vi "GetTransconductanceIntensity.vi"(7 "LabVIEW Web Service Request":refnum<class "Web Request.lvclass">) -> ()   [LabVIEW 2016]
uses:
  <vilib>/wsapi/Web Request.lvclass
  <vilib>/wsapi/NI_WebServices.lvlib
panel:
  # "Use the Web Service Request input terminal to call the VIs on the Web Services palette. Do not remove it from the connector pane unless you don't need access to the palette."
  # "Each additional control wired to the connector pane will be available as an input in the URL. To include an indicator in terminal-mode output (the default setting), it must also be wired to the connector pane."
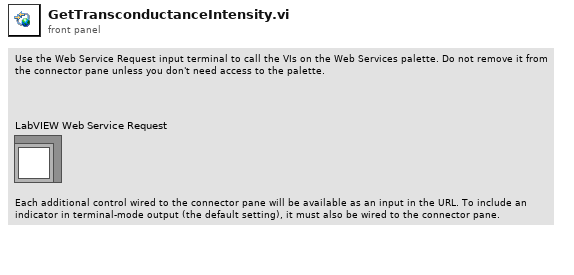
[diagram p1: front panel]
types:
  T1 = typedef "imagedata.ctl" = cluster{"image type":i32, "image depth":i32, "image":u8[], "mask":u8[], "colors":u32[], "Rectangle":cluster{"left":i16, "top":i16, "right":i16, "bottom":i16}}
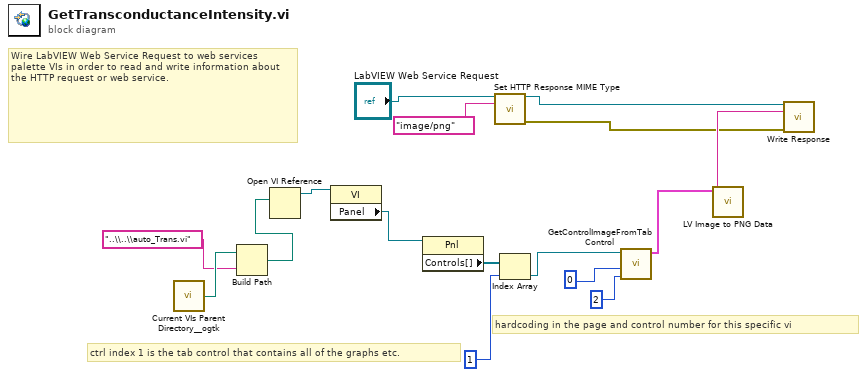
[diagram p0: block diagram]
diagram:
  # "hardcoding in the page and control number for this specific vi"
  # "ctrl index 1 is the tab control that contains all of the graphs etc."
  # "Wire LabVIEW Web Service Request to web services palette VIs in order to read and write information about the HTTP request or web service."
  n1 = call <userlib>:"Current VIs Parent Directory__ogtk.vi"() -> ("Parent Directory (+ Relative)"=w10:path)  [unwired: 5 in]
  n2 = Build Path(base path=w10, name or relative path="..\\..\\auto_Trans.vi") -> (appended path=w8:path)
  n3 = Open VI Reference(vi path=w8) -> (vi reference=w12:refnum<vi>)  [unwired: 5 in, 1 out]
  n4 = property class="VI"(reference=w12) -> ("Panel"=w7:refnum<vi>)  [unwired: 1 in, 2 out]
  n5 = property class="Pnl"(reference=w7) -> ("Controls[]"=w6:refnum<vi>[])  [unwired: 1 in, 2 out]
  n6 = call <vilib>:"Set HTTP Response MIME Type.vi"("LabVIEW Web Service Request"="LabVIEW Web Service Request", "MIME type (text/html)"="image/png") -> ("LabVIEW Web Service Request out"=w15:refnum<class "Web Request.lvclass">, "error out"=w13:errorcluster)  [unwired: 12 in]
  n7 = Index Array(array=w6, index=1) -> (element=w4:refnum<vi>)
  n8 = call "GetControlImageFromTabControl.vi"("page"=2, "control"=0, "Ctl Refnum"=w4) -> ("image data"=w11:T1)  [unwired: 6 in, 2 out]
  n9 = call <vilib>:"LV Image to PNG Data.vi"("image data"=w11) -> ("png data"=w14:string)  [unwired: 9 in, 1 out]
  n10 = call <vilib>:"Write Response.vi"("LabVIEW Web Service Request"=w15, "response string"=w14, "error in (no error)"=w13) -> ()  [unwired: 11 in, 2 out]
